vi "Assert Add Excel Sheets.vi"() -> ()   [LabVIEW 2015]
panel:
  in  "Name":string
  in  "path":path
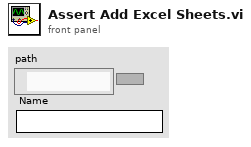
[diagram p1: front panel]
types:
  T1 = cluster{"Excel._Application":refnum<k7>, "Workbooks":refnum<k7>}
  T2 = cluster{"Excel._Application":refnum<k7>, "Workbooks":refnum<k7>, "Open":refnum<k7>}
  T3 = cluster{"Excel._Application":refnum<k7>, "Workbooks":refnum<k7>, "Open":refnum<k7>, "Worksheets":refnum<k7>, "Excel._Worksheet":refnum<k7>}
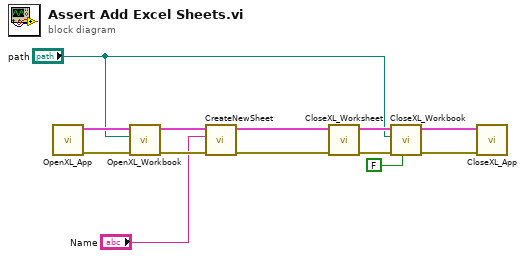
[diagram p0: block diagram]
diagram:
  n1 = call "OpenXL_App.vi"() -> ("error out"=w12:errorcluster, "Refnum Cluster"=w13:T1)  [unwired: 10 in]
  n2 = call "OpenXL_Workbook.vi"("error in"=w12, "path"="path", "Refnum Cluster In"=w13) -> ("error out"=w11:errorcluster, "Refnum Cluster Out"=w9:T2)  [unwired: 7 in]
  n3 = call "CreateNewSheet.vi"("error in (no error)"=w11, "SheetName"="Name", "Refnum Cluster In"=w9) -> ("error out"=w8:errorcluster, "Refnum Cluster Out"=w7:T3)  [unwired: 7 in]
  n4 = call "CloseXL_Worksheet.vi"("error in (no error)"=w8, "Refnum Cluster In"=w7) -> ("error out"=w6:errorcluster, "Refnum Cluster Out"=w5:T2)  [unwired: 8 in]
  n5 = call "CloseXL_Workbook.vi"("Save? (F)"=FALSE, "error in (no error)"=w6, "path"="path", "Refnum Cluster In"=w5) -> ("error out"=w4:errorcluster, "Refnum Cluster Out"=w3:T1)  [unwired: 6 in]
  n6 = call "CloseXL_App.vi"("error in (no error)"=w4, "Refnum Cluster In"=w3) -> ()  [unwired: 9 in, 1 out]
